vi "Create Controls.vi"(0 "vi in":refnum<vi>, 5 "ctl refnum":refnum<vi>, 7 "control label":string, 11 "error in":errorcluster) -> (15 "error out":errorcluster)   [LabVIEW 2021, in "Converter.lvlib"]
uses:
  Converter.lvlib
  <vilib>/numeric/LVNumericRepresentation.ctl
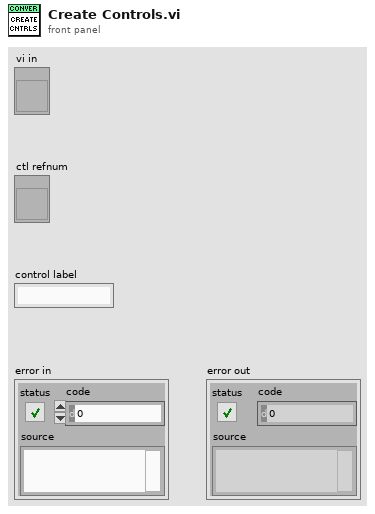
[diagram p1: front panel]
types:
  T1 = typedef "LVNumericRepresentation.ctl" = enum32{"Extended Precision", "Double Precision", "Single Precision", "Long", "Word", "Byte", "Unsigned Long", "Unsigned Word", "Unsigned Byte", "Complex Extended", "Complex Double", "Complex Single", "Quad", "Unsigned Quad", "Fixed-Point"}
  T2 = typedef "LVPositionTypeDef.ctl" = cluster{"Left":i32, "Top":i32}
  T3 = enum32{"not a typedef", "typedef", "strict typedef", "class private data"}
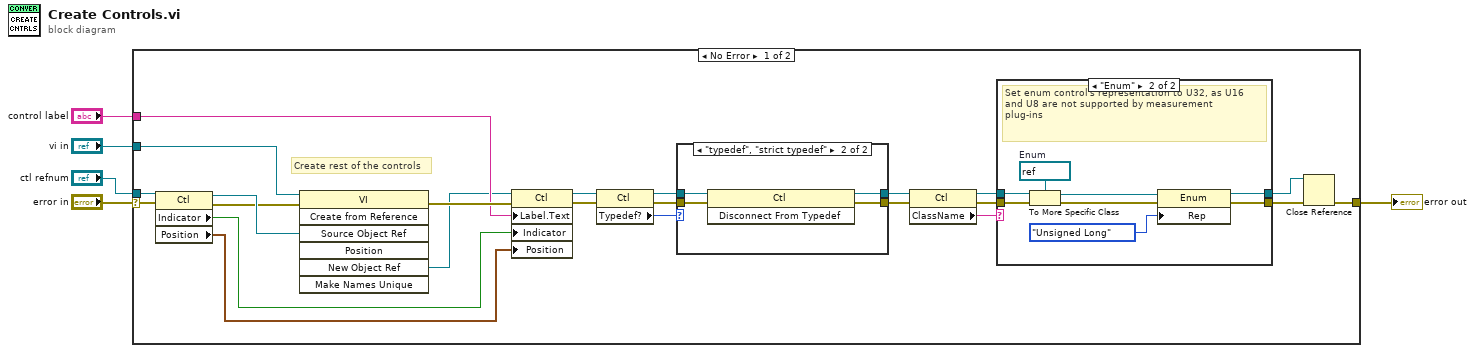
[diagram p0: block diagram]
diagram:
  n1 = case shown="No Error" "error in" {
    selector: "error in" -> [w26 w45]
    tunnel: "ctl refnum" -> [w25 _]
    tunnel: "control label" -> [w23 _]
    tunnel: [w21 w45] -> w1
    tunnel: "vi in" -> [w20 _]
    frame No Error {
      # "Create rest of the controls"
      n2 = property class="Ctl"(reference=w25, error in=w26) -> (reference out=w28:refnum<vi>, error out=w27:errorcluster, "Indicator"=w15:bool, "Position"=w14:T2)
      n3 = invoke class="VI" method="Create from Reference"(reference=w20, error in=w27, "Source Object Ref"=w28) -> (error out=w24:errorcluster, "New Object Ref"=w22:refnum<vi>)  [unwired: 4 in, 5 out]
      n4 = property class="Ctl"(reference=w22, error in=w24, "Label.Text"=w23, "Indicator"=w15, "Position"=w14) -> (reference out=w17:refnum<vi>, error out=w19:errorcluster)
      n5 = property class="Ctl"(reference=w17, error in=w19) -> (reference out=w16:refnum<vi>, error out=w18:errorcluster, "Typedef?"=w13:T3)
      n6 = case shown="\"typedef\", \"strict typedef\"" w13 {
        tunnel: w18 -> [w40 w44]
        tunnel: w16 -> [w39 w43]
        tunnel: [w40 w42] -> w9
        tunnel: [w39 w41] -> w8
        frame "not a typedef", Default {
        }
        frame "typedef", "strict typedef" {
          n7 = invoke class="Ctl" method="Disconnect From Typedef"(reference=w43, error in=w44) -> (reference out=w41:refnum<vi>, error out=w42:errorcluster)  [unwired: 1 in, 1 out]
        }
      }
      n8 = property class="Ctl"(reference=w8, error in=w9) -> (reference out=w10:refnum<vi>, error out=w12:errorcluster, "ClassName"=w11:string)
      n9 = case shown="\"Enum\"" w11 {
        tunnel: [w30 w35] -> w7
        tunnel: w12 -> [w30 w38]
        tunnel: w10 -> [w29 w37]
        tunnel: [w29 w32] -> w6
        frame Default {
        }
        frame "Enum" {
          w33 = refnum<vi> refnum  # Enum
          # "Set enum control's representation to U32, as U16 \nand U8 are not supported by measurement \nplug-ins"
          n10 = To More Specific Class(target class=w33, reference=w37, error in=w38) -> (specific class reference=w34:refnum<vi>, error out=w36:errorcluster)
          n11 = property class="Enum"(reference=w34, error in=w36, "Rep"=LVNumericRepresentation."Unsigned Long" ("Representation")) -> (reference out=w32:refnum<vi>, error out=w35:errorcluster)
        }
      }
      n12 = Close Reference(reference=w6, error in (no error)=w7) -> (error out=w21:errorcluster)
    }
    frame Error {
    }
  }
  "error out" <- w1
